vi "Read Module Error Configurations.vi"(7 "Module ID":string, 8 "error in":errorcluster, 11 "Standard Engine Repo Data in":refnum<class "Standard Engine Configuration.lvclass">) -> (0 "error out":errorcluster, 2 "error responses":T1, 3 "Standard Engine Repo Data out":refnum<class "Standard Engine Configuration.lvclass">)   [LabVIEW 2013, in "Standard Engine Configuration.lvclass"]
doc: "Returns the error configuration for a specific module."
uses:
  Standard Engine Configuration.lvclass
  Runtime/error responses.ctl
  error options.ctl
  Standard Engine Configuration.lvclass/Standard Engine Configuration.ctl
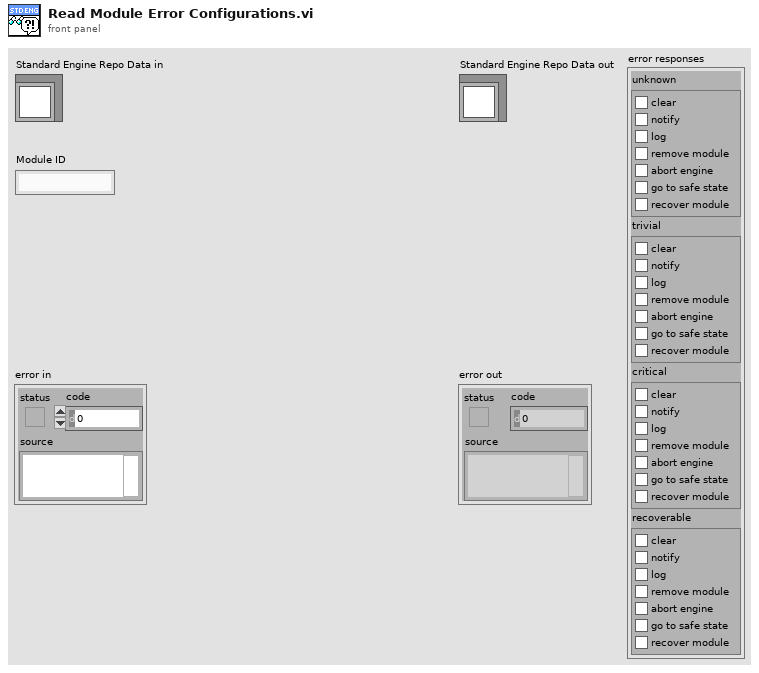
[diagram p1: front panel]
types:
  T1 = typedef "Standard Engine Configuration.lvclass/error responses.ctl" = cluster{"unknown":T2, "trivial":T2, "critical":T2, "recoverable":T2}
  T2 = typedef "Standard Engine Configuration.lvclass/error options.ctl" = cluster{"clear":bool, "notify":bool, "log":bool, "remove module":bool, "abort engine":bool, "go to safe state":bool, "recover module":bool}
  T3 = typedef "Standard Engine Configuration.lvclass/Module Specific Configuration.ctl" = cluster{"Module ID":string, "Module Decimation":T4, "error tag":string, "error responses":T1, "Initialize on Error?":bool}
  T4 = typedef "Standard Engine Configuration.lvclass/Module Decimation.ctl" = cluster{"Decimation":u16, "Offset":u16, "sort order":i32, "async?":bool}
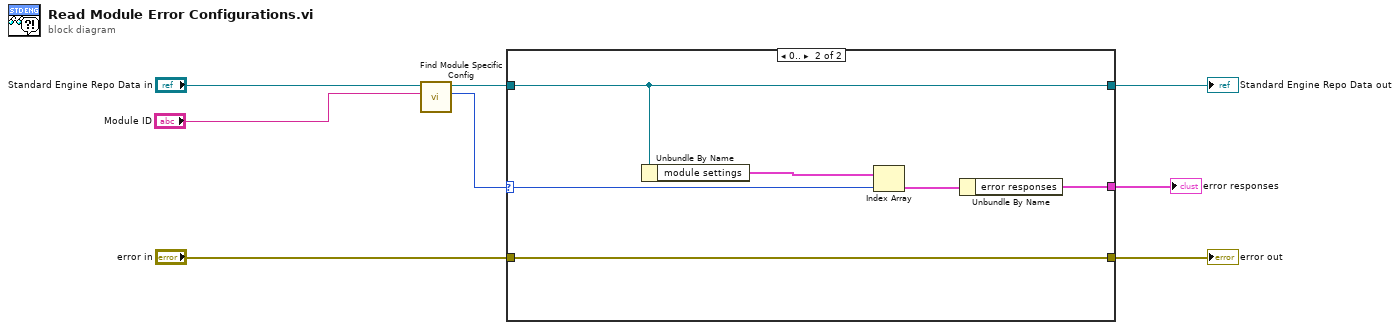
[diagram p0: block diagram]
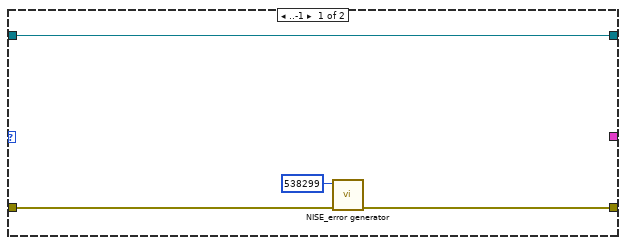
[diagram p2: hidden frame]
diagram:
  n1 = call "Find Module Specific Config.vi"("Module ID"="Module ID", "Standard Engine Repo Data in"="Standard Engine Repo Data in") -> ("Index"=w1:i32, "Standard Engine Repo Data out"=w2:refnum<class "Standard Engine Configuration.lvclass">)  [unwired: 8 in]
  n2 = case shown="0.." w1 {
    selector: w1 -> [_ w14]
    tunnel: w2 -> [w12 w15]
    tunnel: [_ w16] -> w3
    tunnel: "error in" -> [w11 w13]
    tunnel: [w10 w13] -> w6
    tunnel: [w12 w15] -> w4
    frame ..-1 {
      n3 = call <vilib>:"NISE_error generator.vi"("error in"=w11, "error code (0)"=538299) -> ("error out"=w10:errorcluster)  [unwired: 7 in]
    }
    frame 0.. {
      n4 = Unbundle By Name(w15) -> ("module settings"=w18:T3[])
      n5 = Index Array(array=w18, index=w14) -> (element=w17:T3)
      n6 = Unbundle By Name(w17) -> ("error responses"=w16:T1)
    }
  }
  "error out" <- w6
  "Standard Engine Repo Data out" <- w4
  "error responses" <- w3
